vi "Uint16 Get Long.vi"(8 "error in (no error)":errorcluster, 11 "Uint16 DVR in":refnum<data-value>) -> (0 "error out":errorcluster, 2 "I64 out":i64, 3 "Uint16 DVR out":refnum<data-value>)   [LabVIEW 2015, in "MDSplus.lvlib"]
uses:
  <vilib>/MDSplus/Library/MDSplus.lvlib
  <vilib>/MDSplus/Classes/Data_Class/Scalar_Class/Uint16_Class/Uint16.lvclass
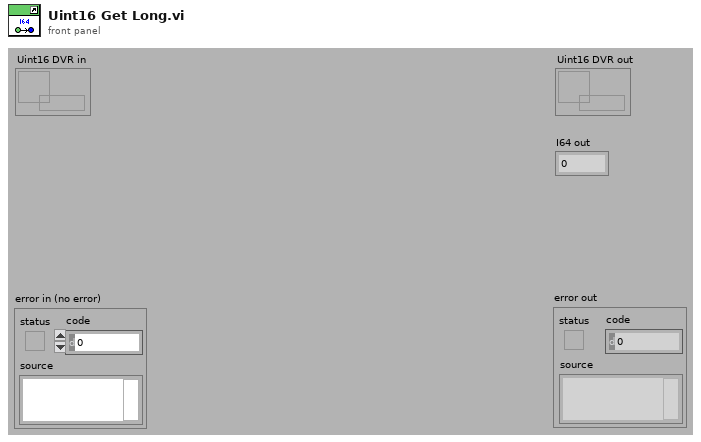
[diagram p1: front panel]
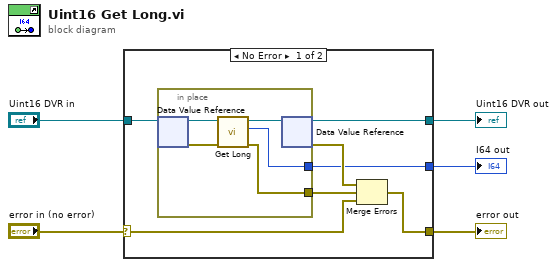
[diagram p0: block diagram]
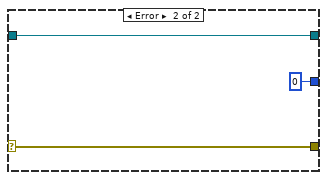
[diagram p2: hidden frame]
diagram:
  n1 = case shown="No Error" "error in (no error)" {
    selector: "error in (no error)" -> [w10 w19]
    tunnel: "Uint16 DVR in" -> [w12 w18]
    tunnel: [w8 w19] -> w5
    tunnel: [w7 w18] -> w1
    tunnel: [w6 i64 0 ("Float out")] -> w4
    frame No Error {
      n2 = in-place {
        in-place-border: [w15] -> w11
        in-place-border: [w13] -> w6
        n3 = in-place-dvr #1(w12) -> (w17:refnum<class "Uint16.lvclass">, w14:errorcluster)
        n4 = call-dynamic "Get Long.vi"("error in (no error)"=w14, "Uint16 in"=w17) -> ("error out"=w15:errorcluster, "I64 out"=w13:i64, "Uint16 out"=w16:refnum<class "Uint16.lvclass">)  [unwired: 7 in]
        n5 = in-place-dvr #1(w16) -> (w7:refnum<data-value>, w9:errorcluster)
      }
      n6 = Merge Errors(w9, w11, w10) -> (w8:errorcluster)
    }
    frame Error {
    }
  }
  "error out" <- w5
  "I64 out" <- w4
  "Uint16 DVR out" <- w1
